vi "FPGA_target_main.vi"() -> ()   [LabVIEW 2014]
doc: "Main VI of the FPGA code. This code implements a pulsed pattern generator on a NI FPGA card, like an PCI-7811R. By this, the timing of an experiment and its experimental procedure can be controlled with a precision down to a few nanoseconds. See the \"blueprints\" in the \"docs\" folder to view the full specifications.\n\nThe main idea is the following. A simple state machine is used to handle the operations states. The data that are uploaded to the FPGA contain commands, pattern data and additional parameters required for some commands. During upload, the data is copied to internal memory of the FPGA. Before the FPGA starts executing commands, the data is copied from the memory to a in internal FIFO. The data in this FIFO is then used during execution of commands in a single-cycle-loop.\n\nmaintainer: Dietrich Beck, d.beck@gsi.de\nauthor: Falk Ziegler\n\nLicense Agreement for this software:\n\nmaintainer: Dietrich Beck, d.beck@gsi.de\nauthor: Falk Ziegler\n\nLicense Agreement for this software:\n\nCopyright (C) 2009\nFalk Ziegler\nInstitut für Physik\nErnst-Moritz-Arndt Universität\nFelix-Hausdorff-Str. 6\n17487 Greifswald\n\nContact: Falk Ziegler, ziegler@physik.uni-greifswald.de\n\nThis program is free software: you can redistribute it and/or modify it under the terms of the GNU General Public License as published by the Free Software Foundation, either version 3 of the License, or (at your option) any later version.\n\nThis program is distributed in the hope that it will be useful, but WITHOUT ANY WARRANTY; without even the implied warranty of MERCHANTABILITY or FITNESS FOR A PARTICULAR PURPOSE. See the GNU General Public License for more details.\n\nYou should have received a copy of the GNU General Public License along with this program. If not, see <http://www.gnu.org/licenses/>.\n\nFor all questions and ideas contact: ziegler@physik.uni-greifswald.de or d.beck@gsi.de\nLast update: 01-Sep-2009"
uses:
  FPGA_target_state_type.ctl
  <vilib>/Platform/TimedLoop/XDataNode/timing_clust.ctl
  <vilib>/Platform/TimedLoop/XDataNode/nitl_modes.ctl
  <vilib>/Platform/TimedLoop/XDataNode/wakeup.ctl
  <vilib>/rvi/Emulation/niFpgaGetClockAttributes.vi
  <vilib>/rvi/Emulation/niFpgaSctlEmulationGetInTimedLoop.vi
  <vilib>/rvi/Emulation/niFpgaEmulationReportErrorSimple.vi
  <vilib>/rvi/Emulation/niFpgaProcessEmulError.vi
  <vilib>/rvi/Emulation/niFpgaCriticalErrorInLSC.vi
  <vilib>/rvi/eio/common/nirviEmuTemplateMethod_errors.vi
  <vilib>/rvi/interface/RandomDataEmulation/niFpgaRandomDataHandleErrors.vi
  <vilib>/rvi/Memory/Memory_Emulation/nirvimemoryEmulation.vi
  <vilib>/rvi/Memory/Memory_Emulation/nirvimemoryFastEmulation.vi
  <vilib>/rvi/DataTransferAndStorage/Container/Common/niFpgaContainerGetUniqueNameForEmu.vi
  <vilib>/rvi/Memory/Memory_Emulation/niFpgaMemoryEmulationCacheClearOnFirstRun.vi
  <vilib>/rvi/Memory/Memory_Emulation/nirvimemoryEmulationManagerCache_MakeExclusive.vi
  <vilib>/rvi/Memory/Memory_Emulation/niFpgaMemoryEmulationValidateCache.vi
  <vilib>/rvi/Memory/Memory_Emulation/nirvimemoryEmulationManagerCache_InsertValue.vi
  <vilib>/Utility/error.llb/Clear Errors.vi
  <vilib>/rvi/Memory/Memory_Emulation/nirvimemoryEmulationManagerCache_ReleaseExclusive.vi
  <vilib>/rvi/Memory/Memory_Emulation/nirvimemoryEmulationManagerCache_GetValue.vi
  <vilib>/rvi/Emulation/niFpgaEmulationIsFPGAContextNoSignature.vi
  <vilib>/rvi/Memory/Memory_Emulation/nirvimemoryEmulationManagerCache_SetValue.vi
  <vilib>/rvi/Emulation/niFpgaSctlEmulationResourceMgr.vi
  <vilib>/Platform/TimedLoop/XDataNode/XDataNode.xnode
  <vilib>/eio/EIONode/EIONode.xnode
  <vilib>/rvi/DataTransferAndStorage/Container/XNode/niFpgaContainer.xnode
  <vilib>/rvi/interface/RandomDataEmulation/nirviRandomDataFpgaReadWriteTemplate.vi
  host/instrumentDriver/NI-FPGA_PPG_Driver.lvlib
  <vilib>/Platform/TimedLoop/XDataNode/XDNodeRunTimeDep.lvlib
panel:
  in  "useJump":bool
  out "ticks_per_us":i32
  out "revision":i32
  in  "query":bool
  out "elements_loaded":i32
  in  "replace":bool
  in  "run":bool
  in  "load":bool
  in  "reset":bool
  in  "mem_addr":u32
  out "error_code":u8
  out "state":T1
  out "number_of_cmds":u32
  out "stop_addr":u32
  in  "stop":bool
  out "start_sctl":bool
  out "fifo_empty":bool
  in  "continuous":bool
  out "stop_sctl":bool
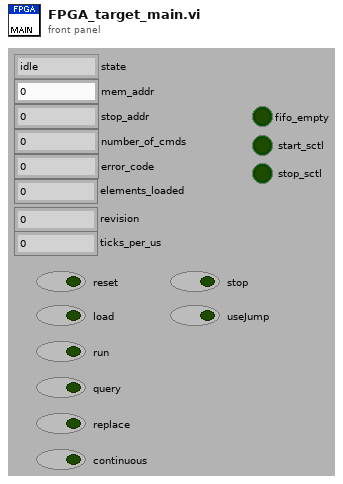
[diagram p1: front panel]
types:
  T1 = typedef "NI-FPGA_PPG_Driver.lvlib/FPGA_target_state_type.ctl" = enum16{"idle", "reset", "query", "load", "run", "stopped"}
  T2 = cluster{"mem_addr":u32, "cmd":u8, "cmd_data":u32}
  T3 = typedef "XDNodeRunTimeDep.lvlib/timing_clust.ctl" = cluster{"Expected End [f-1]":u64, "Actual End [f-1]":u64, "Finished Late? [f-1]":bool, "Expected End [i-1]":u64, "Actual End [i-1]":u64, "Finished Late? [i-1]":bool, "Expected Start [i]":u64, "Actual Start [i]":u64, "Expected Start [f]":u64, "Actual Start [f]":u64, "Source Name":string, "Structure Name":string, "Period":i64, "Deadline":i64, "Offset":i64, "Start":i64, "Priority":i32, "Timeout":i32, "Mode":T4, "Wakeup Reason":T5, "Error":errorcluster, "Source Type":string, "Secondary Source Type":string, "Global End Time":u64, "Global Start Time":u64, "Frame Duration":u64, "Iteration Duration":u64, "Assigned CPU":i32, "I/O Scan Engine Mode":u32}
  T4 = typedef "XDNodeRunTimeDep.lvlib/nitl_modes.ctl" = enum32{"No Change", "Process missed periods, maintain original phase", "Discard missed periods, maintain original phase", "Process missed periods, ignore original phase", "Discard missed periods, ignore original phase"}
  T5 = typedef "XDNodeRunTimeDep.lvlib/wakeup.ctl" = enum32{"Normal", "Aborted", "Asynchronous wakeup", "Timing source error", "Timed loop error", "Timeout"}
  T6 = typedef "FPGA_32BitPattern_data_type.ctl" = cluster{"port0":u8, "port1":u8, "port2":u8, "port3":u8}
  T7 = typedef "FPGA_cmd_data_type.ctl" = cluster{"mem_addr":u32, "cmd":u8, "cmd_data":u32}
  T8 = typedef "FPGA_mem_data_type.ctl" = cluster{"mem_addr":u32, "cmd":u8, "cmd_data":u32, "C0":u32, "C1":u32}
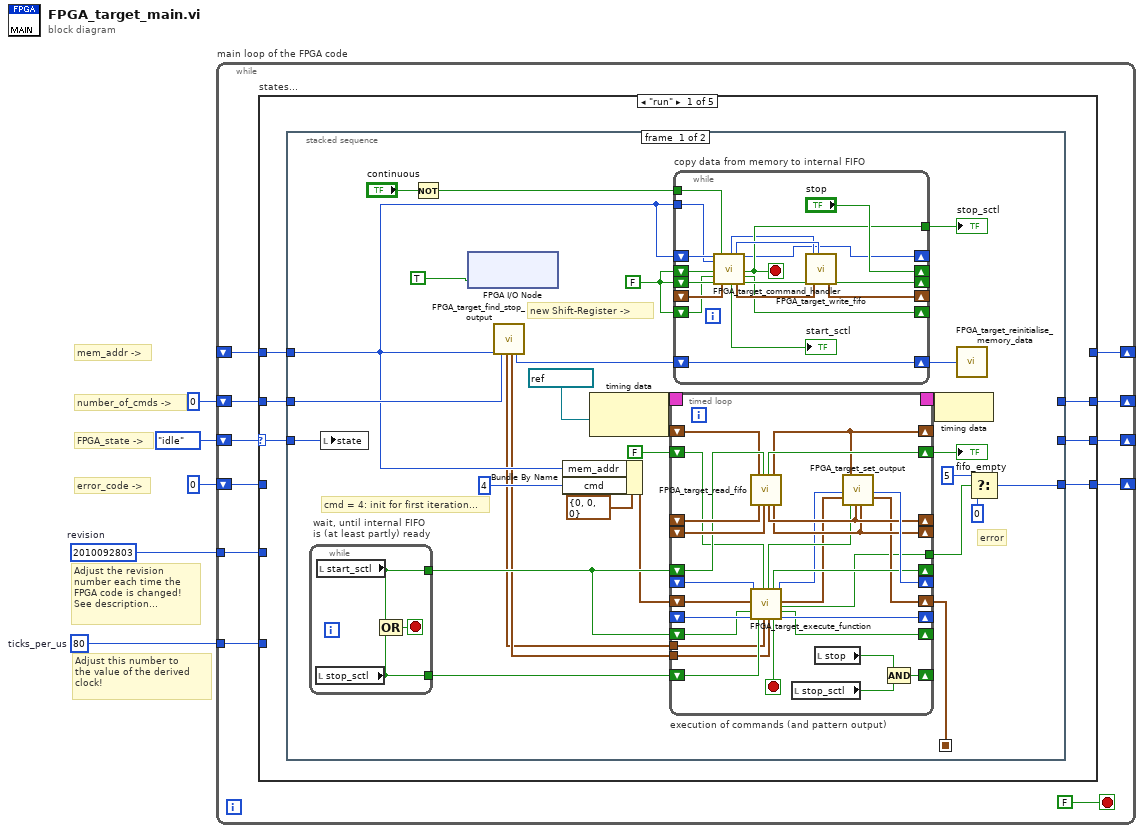
[diagram p0: block diagram]
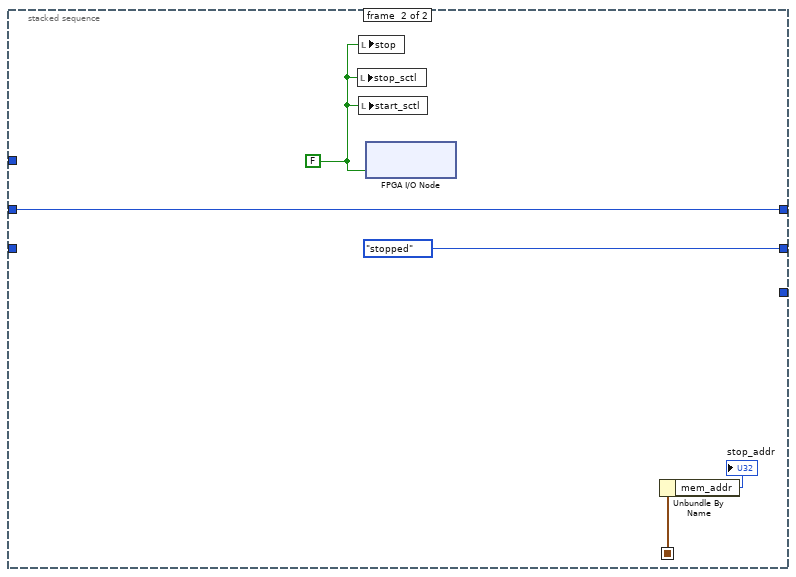
[diagram p2: hidden frame]
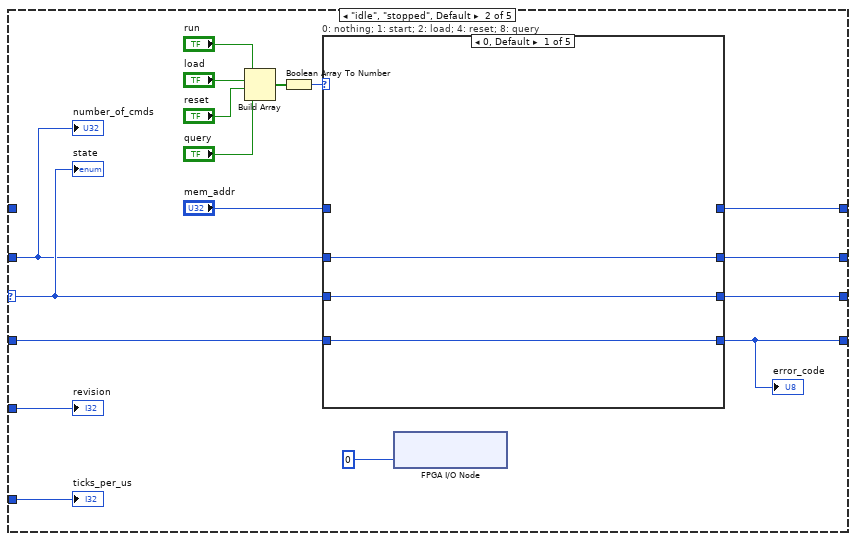
[diagram p3: hidden frame]
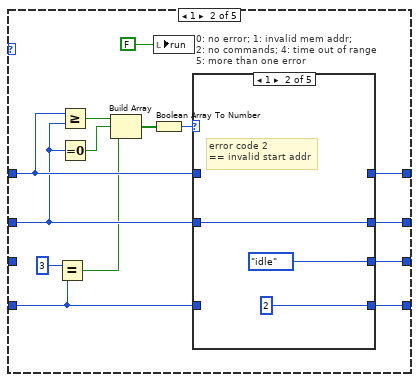
[diagram p4: hidden frame]
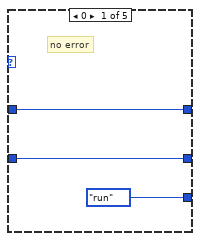
[diagram p5: hidden frame]
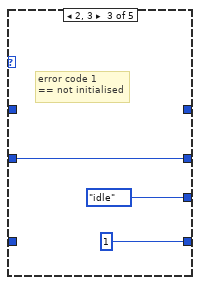
[diagram p6: hidden frame]
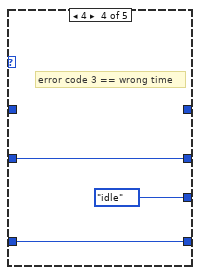
[diagram p7: hidden frame]
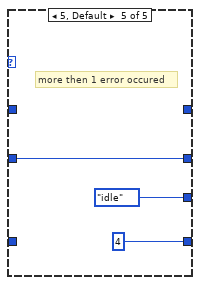
[diagram p8: hidden frame]
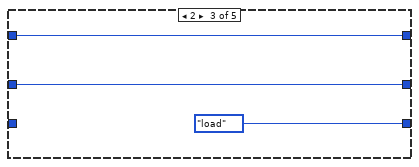
[diagram p9: hidden frame]
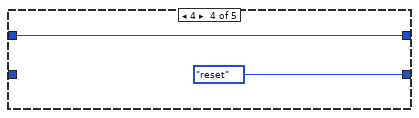
[diagram p10: hidden frame]
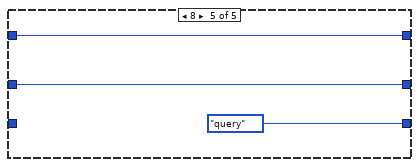
[diagram p11: hidden frame]
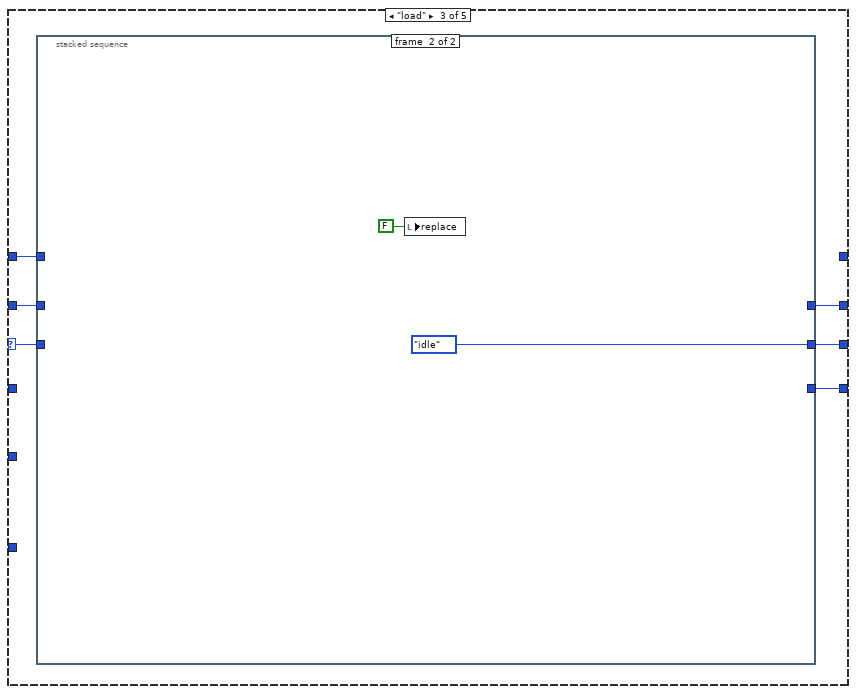
[diagram p12: hidden frame]
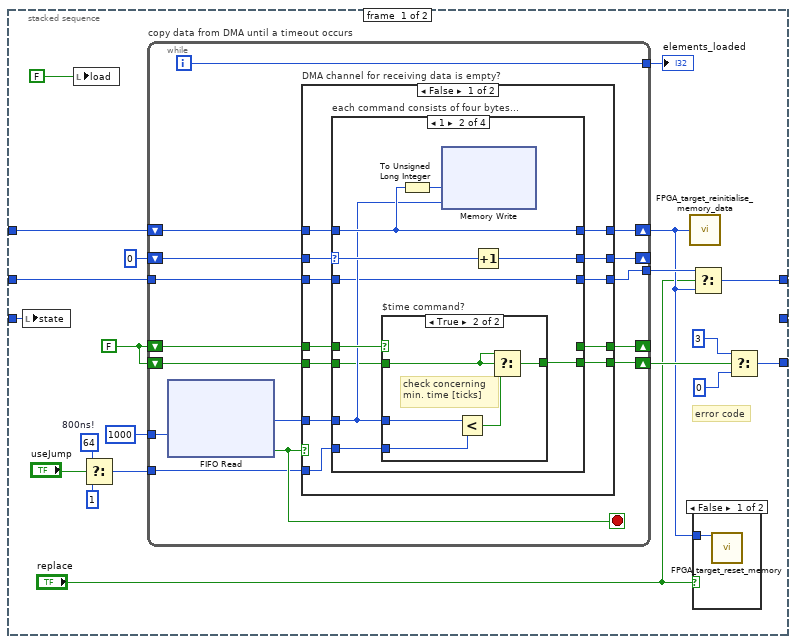
[diagram p13: hidden frame]
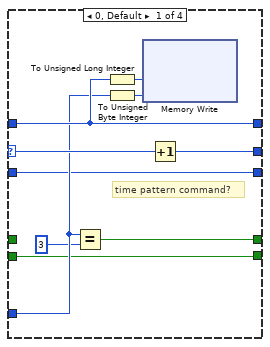
[diagram p15: hidden frame]
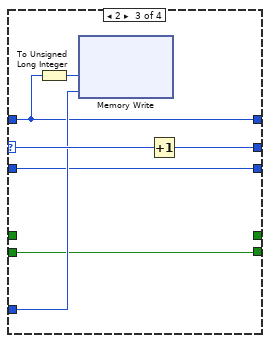
[diagram p17: hidden frame]
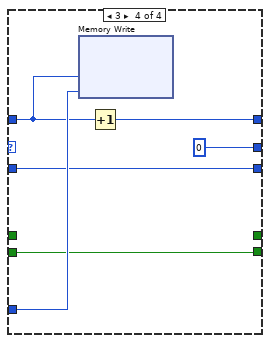
[diagram p18: hidden frame]
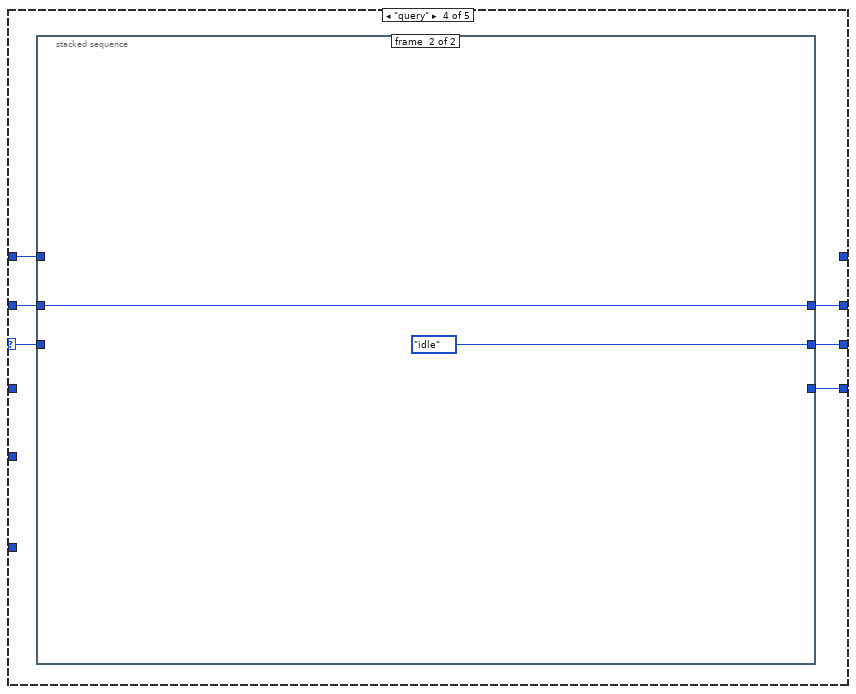
[diagram p20: hidden frame]
diagram:
  w1 = 80  # ticks_per_us
  w2 = 2010092803  # revision
  # "Adjust this number to\nthe value of the derived\nclock!"
  # "Adjust the revision\nnumber each time the\nFPGA code is changed!\nSee description..."
  # "error_code ->"
  # "FPGA_state ->"
  # "number_of_cmds ->"
  # "mem_addr ->"
  n1 = while "main loop of the FPGA code" {
    shift-right: [w14] -> _
    shift-left: FPGA_target_state_type."idle" ("State") -> [w16]
    shift-right: [w13] -> _
    shift-left: _ -> [w12]
    shift-right: [w11] -> _
    shift-left: u8 0 -> [w10]
    shift-right: [w9] -> _
    shift-left: u32 0 ("mem_addr") -> [w8]
    tunnel: w2 -> [w7]
    tunnel: w1 -> [w6]
    stop <- FALSE stop-if-true
    n2 = case "states..." shown="\"run\"" w16 {
      selector: w16 -> [w21 w128 w173 w271 w312]
      tunnel: [w20 w127 w172 w270 FPGA_target_state_type."idle" ("State")] -> w14
      tunnel: [_ w126 _ _ _] -> w13
      tunnel: w12 -> [w22 _ w174 w272 _]
      tunnel: [w17 w114 w170 w268 _] -> w11
      tunnel: w10 -> [_ w125 _ _ _]
      tunnel: [w19 w123 w171 w269 _] -> w9
      tunnel: w8 -> [w18 w124 w169 w267 _]
      tunnel: w7 -> [_ w113 _ _ _]
      tunnel: w6 -> [_ w112 _ _ _]
      frame "run" {
        n3 = stacked-sequence {
          seq-local: [w48 _] -> [_ w109]
          tunnel: w22 -> [w29 _]
          tunnel: w21 -> [w33 _]
          tunnel: [_ FPGA_target_state_type."stopped" ("State")] -> w20
          tunnel: [_ w110] -> w19
          tunnel: w18 -> [w49 w110]
          tunnel: [w47 _] -> w17
          frame #0 {
            w26 = FALSE ("DO_is_active")
            # "cmd = 4: init for first iteration..."
            # "new Shift-Register ->"
            # "error"
            n4 = while "wait, until internal FIFO\nis (at least partly) ready" {
              tunnel: [w105] -> w46
              tunnel: [w104] -> w43
              stop <- w106 stop-if-true
              n5 = local read "stop_sctl"() -> (w105:bool)
              n6 = local read "start_sctl"() -> (w104:bool)
              n7 = Compound Arithmetic op=OR(w104, w105) -> (w106:bool)
            }
            n8 = local write "state"(w33) -> ()
            n9 = Not(x="continuous") -> (.not. x?=w39:bool)
            n10 = xnode "FPGA I/O Node"("DO_state"=TRUE ("DO_is_active")) -> ()  [unwired: 1 in, 1 out]
            n11 = call "FPGA_target_find_stop_output.vi"("start_addr"=w29, "number_cmds_in"=w49) -> ("C0_data"=w27:T6, "C1_data"=w28:T6, "number_cmds_dup"=w40:u32)  [unwired: 14 in, 1 out]
            n12 = Bundle By Name(cluster=T2 {"mem_addr"=0, "cmd"=0, "cmd_data"=0} ("data_out"), "mem_addr"=w29, "cmd"=u8 4) -> (w37:T2)
            n13 = node-c288(refnum<k21> "80MHz" ("Source Name")) -> (w25:T3)
            n14 = timed-loop "execution of commands (and pattern output)" {
              shift-right: [w59] -> _
              shift-left: _ -> [w58]
              shift-right: [w75] -> _
              shift-left: _ -> [w78]
              shift-right: [w74] -> _
              shift-left: _ -> [w77]
              shift-right: [w76] -> _
              shift-left: _ -> [w67]
              shift-right: [w71] -> _
              shift-left: w43 -> [w68]
              shift-right: [w50] -> _
              shift-left: w46 -> [w73]
              shift-right: [w70] -> w45
              shift-left: FALSE ("fifo_empty") -> [w54]
              shift-right: [w56] -> w48
              shift-left: w37 -> [w55]
              shift-right: [w65] -> _
              shift-left: _ -> [w64]
              tunnel: w27 -> [w63]
              tunnel: w28 -> [w62]
              shift-right: [w60] -> _
              shift-left: w43 -> [w61]
              tunnel: [w53] -> w36
              timing: w25 -> [_]
              timing-out: [_] -> w24
              stop <- w69 stop-if-true
              n15 = call "FPGA_target_read_fifo.vi"("data_in"=w58, "C0_in"=w78, "read_fifo"=w68, "C1_in"=w77) -> ("fifo_empty"=w70:bool, "C0_out"=w75:T6, "data_out"=w59:T7, "C1_out"=w74:T6)  [unwired: 12 in]
              n16 = call "FPGA_target_execute_function.vi"("tick_count_in"=w67, "data_in"=w55, "set_stop_output_in"=w61, "input_data_in"=w64, "stop_request"=w73, "fifo_empty_in"=w54, "C0_data"=w63, "C1_data"=w62) -> ("set_output"=w72:bool, "read_fifo"=w71:bool, "stop"=w69:bool, "tick_count_out"=w66:u32, "data_dup"=w57:T7, "fifo_empty_out"=w53:bool, "set_stop_output_out"=w60:bool, "input_data_out"=w65:u8)  [unwired: 4 in]
              n17 = local read "stop_sctl"() -> (w52:bool)
              n18 = local read "stop"() -> (w51:bool)
              n19 = call "FPGA_target_set_output.vi"("tick_count_in"=w66, "data_in"=w57, "new_data_in"=w59, "set_outputs"=w72, "C0_data"=w75, "C1_data"=w74) -> ("tick_count_out"=w76:u32, "data_out"=w56:T7)  [unwired: 12 in]
              n20 = Compound Arithmetic op=AND(w51, w52) -> (w50:bool)
            }
            "fifo_empty" <- w45
            n21 = while "copy data from memory to internal FIFO" {
              shift-right: [w94] -> _
              shift-left: _ -> [w93]
              tunnel: w29 -> [w88]
              tunnel: w39 -> [w90]
              shift-right: [w103] -> w42
              shift-left: w40 -> [w103]
              shift-right: [w92] -> _
              shift-left: w26 -> [w101]
              shift-right: ["stop"] -> _
              shift-left: w26 -> [w96]
              shift-right: [w87] -> _
              shift-left: w29 -> [w97]
              tunnel: [w91] -> w32
              shift-right: [w85] -> _
              shift-left: w26 -> [w86]
              stop <- w91 stop-if-true
              n22 = call "FPGA_target_command_handler.vi"("mem_addr_in"=w97, "mem_addr_start"=w88, "force_stop"=w96, "stop_execution_in"=w86, "FIFO_full"=w101, "continuous"=w90, "mem_data_in"=w93) -> ("mem2_addr"=w89:u32, "start_sctl"=→"start_sctl":bool, "mem2_data"=w98:u32, "mem_data_out"=w95:T8, "mem_addr_ out"=w87:u32, "stop_execution_out"=w91:bool, "stop_triggered"=w85:bool, "write_FIFO"=w102:bool)  [unwired: 5 in]
              n23 = call "FPGA_target_write_fifo.vi"("write_FIFO"=w102, "mem2_addr_in"=w89, "mem_data_in"=w95, "mem2_data"=w98) -> ("mem_data_dup"=w94:T8, "FIFO_full"=w92:bool)  [unwired: 13 in, 1 out]
            }
            "stop_sctl" <- w32
            n24 = node-c288(w24) -> ()
            n25 = call "FPGA_target_reinitialise_memory_data.vi"("number_cmds"=w42) -> ()
            n26 = Select(t=u8 5, s=w36, f=u8 0) -> (s? t:f=w47:u8)
          }
          frame #1 {
            w107 = FALSE ("DO_is_active")
            n27 = local write "stop_sctl"(w107) -> ()
            n28 = local write "stop"(w107) -> ()
            n29 = local write "start_sctl"(w107) -> ()
            n30 = xnode "FPGA I/O Node"("DO_state"=w107) -> ()  [unwired: 1 in, 1 out]
            n31 = Unbundle By Name(w109) -> ("mem_addr"=→"stop_addr":u32)
          }
        }
      }
      frame "idle", "stopped", Default {
        n32 = Build Array("run", "load", "reset", "query") -> (w118:bool[])
        n33 = Boolean Array To Number(Boolean array=w118) -> (number=w119:u8)
        n34 = case "0: nothing; 1: start; 2: load; 4: reset; 8: query" shown="0, Default" w119 {
          tunnel: [w131 w145 FPGA_target_state_type."load" ("state") FPGA_target_state_type."reset" ("state") FPGA_target_state_type."query" ("state")] -> w127
          tunnel: [_ w139 w162 _ w166] -> w126
          tunnel: "mem_addr" -> [_ w140 w162 _ w166]
          tunnel: w128 -> [w131 _ _ _ _]
          tunnel: [w130 w136 _ _ _] -> w114
          tunnel: w125 -> [w130 w133 _ _ _]
          tunnel: w124 -> [w129 w138 w161 w164 w167]
          tunnel: [w129 w137 w161 w164 w167] -> w123
          frame 0, Default {
          }
          frame 1 {
            n35 = Equal?(x=u8 3 ("y"), y=w133) -> (x = y?=w135:bool)
            n36 = Greater Or Equal?(x=w140, y=w138) -> (x >= y?=w144:bool)
            n37 = Equal To 0?(x=w138) -> (x = 0?=w143:bool)
            n38 = Build Array(w144, w143, w135) -> (w142:bool[])
            n39 = local write "run"(FALSE) -> ()
            n40 = Boolean Array To Number(Boolean array=w142) -> (number=w141:u8)
            n41 = case "0: no error; 1: invalid mem addr; \n2: no commands; 4: time out of range\n5: more than one error" shown="1" w141 {
              tunnel: [FPGA_target_state_type."run" ("state") FPGA_target_state_type."idle" ("state") FPGA_target_state_type."idle" ("state") FPGA_target_state_type."idle" ("state") FPGA_target_state_type."idle" ("state")] -> w145
              tunnel: w140 -> [w147 _ _ _ _]
              tunnel: [w147 _ _ _ _] -> w139
              tunnel: w138 -> [w146 w150 w153 w157 w160]
              tunnel: [w146 w150 w153 w157 w160] -> w137
              tunnel: [_ u8 2 u8 1 w155 u8 4 ("f")] -> w136
              tunnel: w133 -> [_ _ _ w155 _]
              frame 0 {
                # "no error"
              }
              frame 1 {
                # "error code 2 \n== invalid start addr"
              }
              frame 2, 3 {
                # "error code 1 \n== not initialised"
              }
              frame 4 {
                # "error code 3 == wrong time"
              }
              frame 5, Default {
                # "more then 1 error occured"
              }
            }
          }
          frame 2 {
          }
          frame 4 {
          }
          frame 8 {
          }
        }
        "error_code" <- w114
        n42 = xnode "FPGA I/O Node"("TriggerIn_0-7"=u8 0 ("DI_port0")) -> ()  [unwired: 1 in, 1 out]
        "state" <- w128
        "number_of_cmds" <- w124
        "revision" <- w113
        "ticks_per_us" <- w112
      }
      frame "load" {
        n43 = stacked-sequence {
          tunnel: w174 -> [w180 _]
          tunnel: w173 -> [w193 _]
          tunnel: [_ FPGA_target_state_type."idle" ("State")] -> w172
          tunnel: [w184 _] -> w171
          tunnel: [w187 _] -> w170
          tunnel: w169 -> [w186 _]
          frame #0 {
            w175 = u32 64  # 800ns!
            w191 = FALSE
            # "error code"
            n44 = local write "state"(w193) -> ()
            n45 = local write "load"(FALSE ("load")) -> ()
            n46 = Select(t=w175, s="useJump", f=u32 1 ("x")) -> (s? t:f=w176:u32)
            n47 = while "copy data from DMA until a timeout occurs" {
              tunnel: 1000 -> [w205]
              shift-right: [w206] -> _
              shift-left: u16 0 -> [w209]
              shift-right: [w207] -> w183
              shift-left: w180 -> [w208]
              shift-right: [w202] -> _
              shift-left: w191 -> [w203]
              shift-right: [w200] -> w190
              shift-left: w191 -> [w201]
              tunnel: w186 -> [w199]
              tunnel: [w198] -> w185
              tunnel: [w197] -> w179
              tunnel: w176 -> [w196]
              i -> [w197]
              stop <- w204 stop-if-true
              n48 = xnode ("FIFO Read")("Timeout"=w205) -> ("Element"=w210:u32, "Timed Out?"=w204:bool)  [unwired: 1 in, 1 out]
              n49 = case "DMA channel for receiving data is empty?" shown="False" w204 {
                tunnel: w210 -> [w221 _]
                tunnel: w209 -> [w222 _]
                tunnel: w208 -> [w220 w264]
                tunnel: [w218 w264] -> w207
                tunnel: [w219 _] -> w206
                tunnel: w203 -> [w217 _]
                tunnel: [w216 _] -> w202
                tunnel: w201 -> [w215 w263]
                tunnel: [w214 w263] -> w200
                tunnel: w199 -> [w213 w262]
                tunnel: [w212 w262] -> w198
                tunnel: w196 -> [w211 _]
                frame False {
                  n50 = case "each command consists of four bytes..." shown="1" w222 {
                    selector: w222 -> [w232 w242 w255 _]
                    tunnel: w221 -> [w226 w237 w253 w259]
                    tunnel: w220 -> [w229 w239 w251 w258]
                    tunnel: [w229 w239 w251 w260] -> w218
                    tunnel: [w231 w241 w254 u16 0] -> w219
                    tunnel: w217 -> [_ w238 _ _]
                    tunnel: [w227 _ _ _] -> w216
                    tunnel: w215 -> [w224 w236 w250 w257]
                    tunnel: [w224 w235 w250 w257] -> w214
                    tunnel: w213 -> [w223 w234 w249 w256]
                    tunnel: [w223 w234 w249 w256] -> w212
                    tunnel: w211 -> [_ w233 _ _]
                    frame 0, Default {
                      # "time pattern command?"
                      n51 = Equal?(x=w226, y=u32 3 ("x")) -> (x = y?=w227:bool)
                      n52 = To Unsigned Long Integer(number=w229) -> (unsigned 32bit integer=w230:u32)
                      n53 = To Unsigned Byte Integer(number=w226) -> (unsigned 8bit integer=w228:u8)
                      n54 = xnode ("Memory Write")("Address"=w230, "Data"=w228) -> ()  [unwired: 1 in, 1 out]
                      n55 = Increment(x=w232) -> (x+1=w231:u16)
                    }
                    frame 1 {
                      n56 = case "$time command?" shown="True" w238 {
                        tunnel: w237 -> [_ w247]
                        tunnel: w236 -> [w243 w248]
                        tunnel: [w243 w245] -> w235
                        tunnel: w233 -> [_ w244]
                        frame False {
                        }
                        frame True {
                          # "check concerning\nmin. time [ticks]"
                          n57 = Less?(x=w247, y=w244) -> (x < y?=w246:bool)
                          n58 = Select(t=w248, s=w248, f=w246) -> (s? t:f=w245:bool)
                        }
                      }
                      n59 = To Unsigned Long Integer(number=w239) -> (unsigned 32bit integer=w240:u32)
                      n60 = xnode ("Memory Write")("Address"=w240, "Data"=w237) -> ()  [unwired: 1 in, 1 out]
                      n61 = Increment(x=w242) -> (x+1=w241:u16)
                    }
                    frame 2 {
                      n62 = To Unsigned Long Integer(number=w251) -> (unsigned 32bit integer=w252:u32)
                      n63 = xnode ("Memory Write")("Address"=w252, "Data"=w253) -> ()  [unwired: 1 in, 1 out]
                      n64 = Increment(x=w255) -> (x+1=w254:u16)
                    }
                    frame 3 {
                      n65 = xnode ("Memory Write")("Address"=w258, "Data"=w259) -> ()  [unwired: 1 in, 1 out]
                      n66 = Increment(x=w258) -> (x+1=w260:u32)
                    }
                  }
                }
                frame True {
                }
              }
            }
            "elements_loaded" <- w179
            n67 = call "FPGA_target_reinitialise_memory_data.vi"("number_cmds"=w183) -> ()
            n68 = Select(t=w185, s="replace", f=w183) -> (s? t:f=w184:u32)
            n69 = case shown="False" "replace" {
              tunnel: w183 -> [w195 _]
              frame False {
                n70 = call "FPGA_target_reset_memory.vi"("mem_addr_in"=w195) -> ()  [unwired: 18 in, 1 out]
              }
              frame True {
              }
            }
            n71 = Select(t=u8 3, s=w190, f=u8 0) -> (s? t:f=w187:u8)
          }
          frame #1 {
            n72 = local write "replace"(FALSE ("replace")) -> ()
          }
        }
      }
      frame "query" {
        n73 = stacked-sequence {
          tunnel: w272 -> [w283 _]
          tunnel: w271 -> [_ _]
          tunnel: [_ FPGA_target_state_type."idle" ("State")] -> w270
          tunnel: [_ w307] -> w269
          tunnel: [w273 _] -> w268
          tunnel: w267 -> [_ w307]
          frame #0 {
            # "error"
            n74 = local write "query"(FALSE ("load")) -> ()
            n75 = call "FPGA_target_read_memory.vi"("addr_in"=w283) -> ("data_mem0"=w282:u8, "data_mem1"=w280:u32, "data_mem2"=w279:u32, "data_mem3"=w281:u32, "addr_dup"=w278:u32)  [unwired: 13 in, 1 out]
            n76 = while "for all bytes of a command" {
              tunnel: w282 -> [w293]
              tunnel: w281 -> [w292]
              tunnel: w280 -> [w291]
              tunnel: w279 -> [w290]
              tunnel: w278 -> [_]
              tunnel: 3 -> [w288]
              tunnel: [w285] -> w276
              i -> [w289]
              stop <- w286 stop-if-true
              n77 = Equal?(x=w289, y=w288) -> (x = y?=w287:bool)
              n78 = case "each command has four bytes..." shown="0, Default" w289 {
                tunnel: w293 -> [w297 _ _ _]
                tunnel: [w294 w299 w302 w305] -> w285
                tunnel: w292 -> [_ w298 _ _]
                tunnel: w291 -> [_ _ w301 _]
                tunnel: w290 -> [_ _ _ w304]
                frame 0, Default {
                  n79 = To Unsigned Long Integer(number=w297) -> (unsigned 32bit integer=w296:u32)
                  n80 = xnode ("FIFO Write")("Element"=w296, "Timeout"=0) -> ("Timed Out?"=w294:bool)  [unwired: 1 in, 1 out]
                }
                frame 1 {
                  n81 = xnode ("FIFO Write")("Element"=w298, "Timeout"=0) -> ("Timed Out?"=w299:bool)  [unwired: 1 in, 1 out]
                }
                frame 2 {
                  n82 = xnode ("FIFO Write")("Element"=w301, "Timeout"=0) -> ("Timed Out?"=w302:bool)  [unwired: 1 in, 1 out]
                }
                frame 3 {
                  n83 = xnode ("FIFO Write")("Element"=w304, "Timeout"=0) -> ("Timed Out?"=w305:bool)  [unwired: 1 in, 1 out]
                }
              }
              n84 = Compound Arithmetic op=OR(w285, w287) -> (w286:bool)
            }
            n85 = Select(t=u8 6, s=w276, f=u8 0) -> (s? t:f=w273:u8)
          }
          frame #1 {
          }
        }
      }
      frame "reset" {
        w309 = FALSE ("reset")
        n86 = local write "continuous"(w309) -> ()
        n87 = local write "reset"(w309) -> ()
        n88 = local write "state"(w312) -> ()
        n89 = call "FPGA_target_reset_memory.vi"("mem_addr_in"=u32 0) -> ()  [unwired: 18 in, 1 out]
      }
    }
  }
